vi "MasterVI-Blank.vi"() -> ()   [LabVIEW 2011]
panel:
  out "SubVI Results":dbl[][](graph)
  out "A and B":dbl[][](graph)
  in  "Signal Specs":T1(array[cluster]) {"phase" format="%0.2f"; "dc offset" format="%0.2f"; "amplitude" format="%0.2f"; "frequency" format="%0.2f"}
  in  "# of samples":i32=100
  # "A"
  # "B"
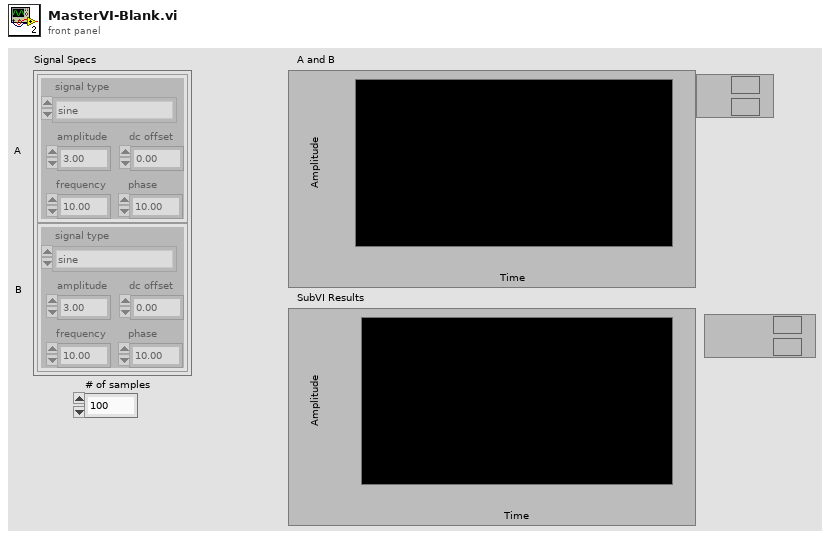
[diagram p1: front panel]
types:
  T1 = cluster{"signal type":enum16{"sine", "cosine", "triangle", "square", "sawtooth", "increasing ramp", "decreasing ramp"}, "frequency":dbl, "amplitude":dbl, "dc offset":dbl, "phase":dbl}[]
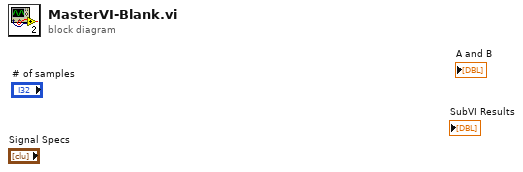
[diagram p0: block diagram]
diagram:
